vi "magboard_128_calibrate_nodes.vi"(11 "Sensor Input (mT)":dbl[][](array[numeric])) -> (3 "Sensor Output - Position (mm)":dbl[][](array[numeric]))   [LabVIEW 2018]
uses:
  FGVs/FGV States.ctl
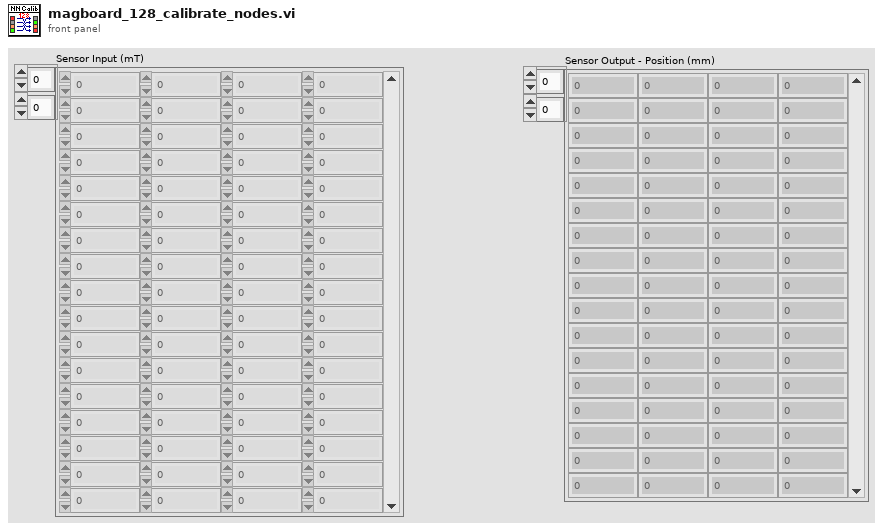
[diagram p1: front panel]
types:
  T1 = typedef "FGV States.ctl" = enum16{"Get", "Set", "Reset"}
  T2 = cluster{cluster{dbl[][], "Array":dbl[][]}, cluster{dbl[][], "Array":dbl[][]}, cluster{dbl[][], "Array":dbl[][]}, cluster{dbl[][], "Array":dbl[][]}}[]
  T3 = cluster{cluster{dbl[][], "Array":dbl[][]}, cluster{dbl[][], "Array":dbl[][]}, cluster{dbl[][], "Array":dbl[][]}, cluster{dbl[][], "Array":dbl[][]}}
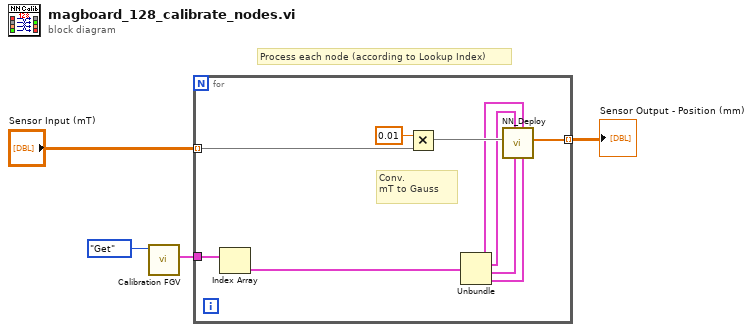
[diagram p0: block diagram]
diagram:
  # "Process each node (according to Lookup Index)"
  n1 = call "Calibration FGV.vi"("FGV States"=FGV_States."Get") -> ("Calib in 2"=w3:T2)  [unwired: 10 in]
  n2 = for {
    tunnel: w3 -> [w7]
    tunnel: [w8] -> w2 mode=indexing
    tunnel: "Sensor Input (mT)" -> [w5] mode=indexing
    # "Conv. \nmT to Gauss"
    n3 = Index Array(array=w7) -> (element=w6:T3)  [unwired: 1 in]
    n4 = Multiply(x=0.01, y=w5) -> (x*y=w13:dbl[])
    n5 = Unbundle(w6) -> (w12:cluster{dbl[][], "Array":dbl[][]}, w11:cluster{dbl[][], "Array":dbl[][]}, w10:cluster{dbl[][], "Array":dbl[][]}, w9:cluster{dbl[][], "Array":dbl[][]})
    n6 = call "NN_Deploy.vi"("Output Layer"=w9, "Input Layer"=w12, "Layer 2"=w10, "Layer 1"=w11, "Input"=w13) -> ("Output"=w8:dbl[])  [unwired: 6 in]
  }
  "Sensor Output - Position (mm)" <- w2
